vi "fp5YES.vi"   [LabVIEW 2016]
uses:
  <vilib>/NXT/Block Support/NXT_OutputPort.ctl
  <vilib>/NXT/Block Support/NXT_InputPort.ctl
  <vilib>/NXT/NXTIO Xnodes/NXTIONodeSubVIs/LEGOResetMotors.vi
  <vilib>/NXT/Dual Mode Library/Sensors/Touch_Released.vi
  <vilib>/NXT/Dual Mode Library/Sensors/EV3_Color_Reflect.vi
  <vilib>/NXT/NXTIO Xnodes/NXTIONodeSubVIs/NXTMoveMotors.vi
  <vilib>/NXT/NXTIO Xnodes/NXTIONodeSubVIs/NXTMotorRunDistance.vi
  <vilib>/NXT/NXTIO Xnodes/NXTIONodeSubVIs/NXTStopMotors.vi
  <vilib>/NXT/Dual Mode Library/Sound/PlayAsharp.vi
  <vilib>/NXT/Dual Mode Library/Sound/PlayC.vi
  <vilib>/NXT/Subs/LVHSConnector.ctl
  <vilib>/NXT/NXTIO Xnodes/AddressXNode/NXTIOAddress.xnode
  <vilib>/NXT/NXTIO Xnodes/NXTIOXNode/NXTIO.xnode
  <vilib>/NXT/LegoClasses/BrickReference/BrickReference.lvclass
types:
  T1 = typedef "NXT_OutputPort.ctl" = u8
  T2 = typedef "NXT_InputPort.ctl" = u32
  T3 = typedef "LVHSConnector.ctl" = refnum<class "BrickReference.lvclass">
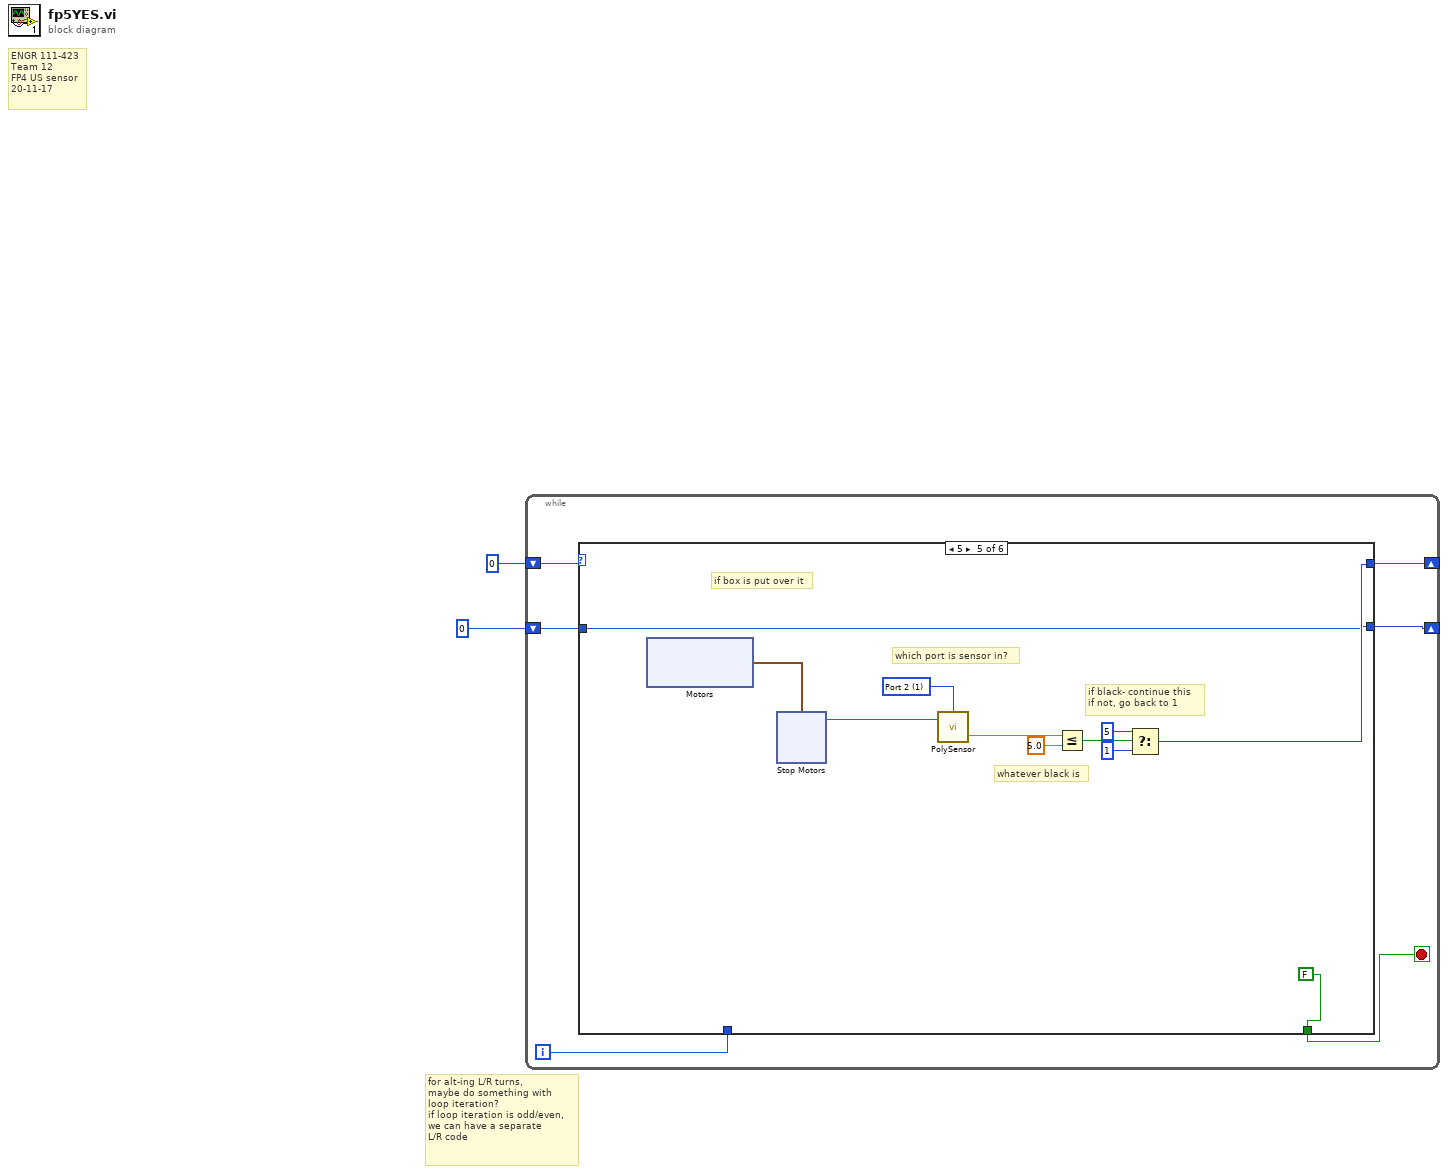
[diagram p0: block diagram]
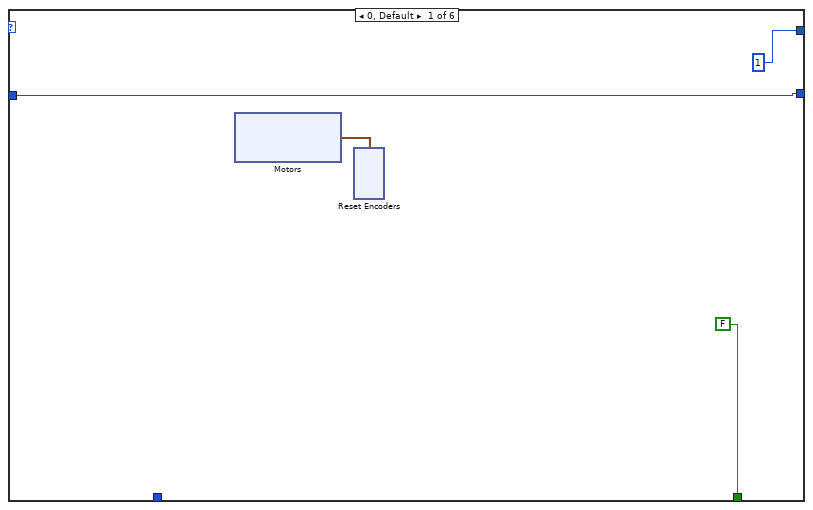
[diagram p2: hidden frame]
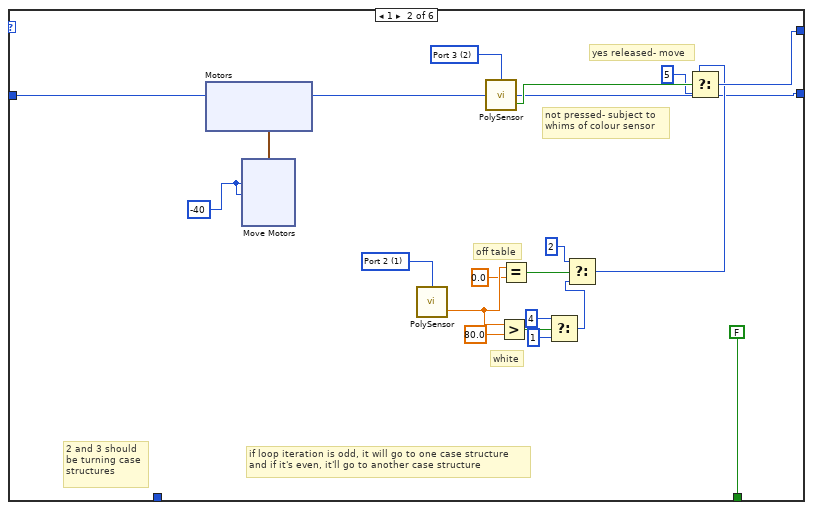
[diagram p3: hidden frame]
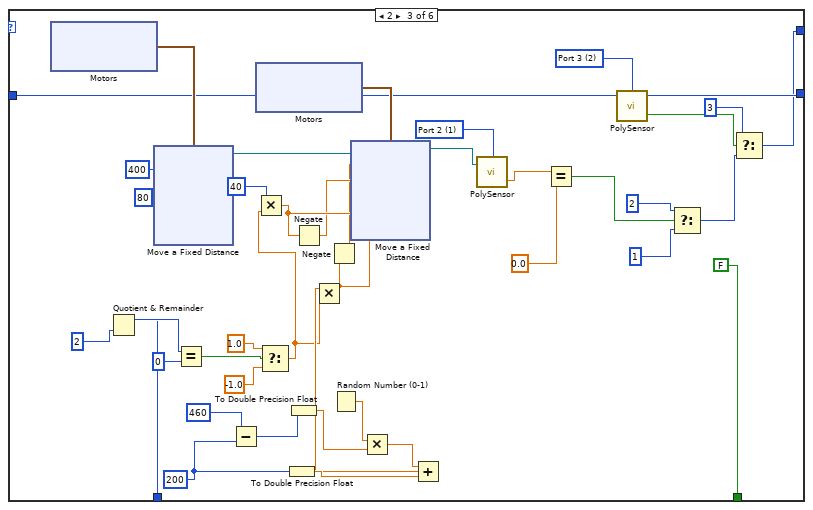
[diagram p4: hidden frame]
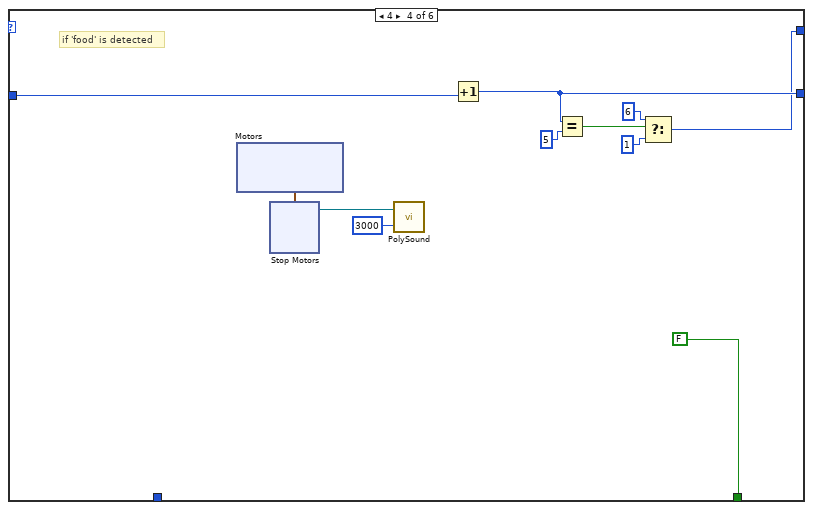
[diagram p5: hidden frame]
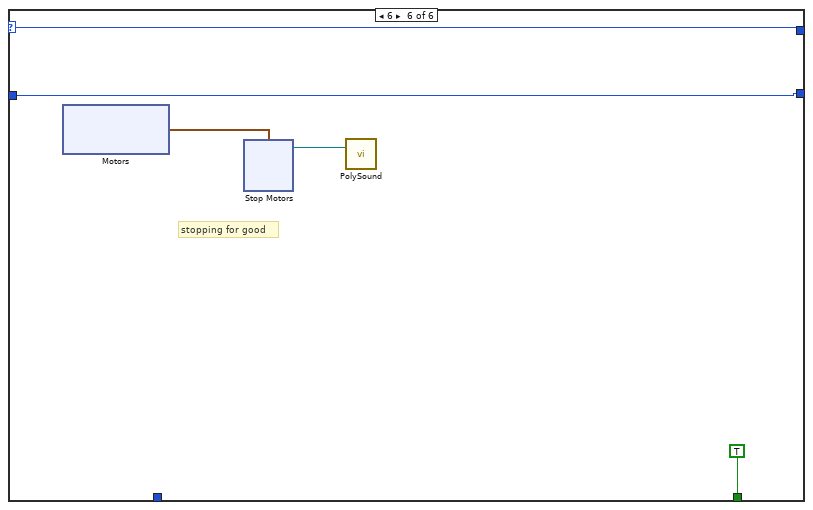
[diagram p6: hidden frame]
diagram:
  # "for alt-ing L/R turns,\nmaybe do something with\nloop iteration?\nif loop iteration is odd/even,\nwe can have a separate\nL/R code"
  # "ENGR 111-423\nTeam 12\nFP4 US sensor\n20-11-17"
  n1 = while {
    shift-right: [w6] -> _
    shift-left: 0 -> [w8]
    shift-right: [w4] -> _
    shift-left: 0 -> [w5]
    i -> [w3]
    stop <- w7 stop-if-true
    n2 = case shown="5" w8 {
      selector: w8 -> [_ _ _ _ _ w149]
      tunnel: [FALSE FALSE FALSE FALSE FALSE TRUE] -> w7
      tunnel: [1 w25 w56 w112 w131 w149] -> w6
      tunnel: w5 -> [w9 w19 w57 w119 w129 w146]
      tunnel: [w9 w19 w57 w116 w129 w146] -> w4
      tunnel: w3 -> [_ _ w58 _ _ _]
      frame 0, Default {
        n3 = xnode "Motors"() -> ("Motor"=w10:cluster{"Port":T1, "Port":T1})
        n4 = xnode "Reset Encoders"("Motors"=w10) -> ()  [unwired: 1 in, 1 out]
      }
      frame 1 {
        w26 = T2 1 items=["Port 1", "Port 2", "Port 3", "Port 4"] ("Port (Port 1)")
        w34 = T2 2 items=["Port 1", "Port 2", "Port 3", "Port 4"] ("Port (Port 1)")
        w35 = -40 ("Distance 1")
        # "white"
        # "off table"
        # "2 and 3 should\nbe turning case\nstructures"
        # "if loop iteration is odd, it will go to one case structure\nand if it's even, it'll go to another case structure"
        # "not pressed- subject to\nwhims of colour sensor"
        # "yes released- move"
        n5 = xnode "Motors"() -> ("Motor"=w36:cluster{"Port":T1, "Port":T1})
        n6 = xnode "Move Motors"("Power/Speed 2"=w35, "Power/Speed 1"=w35, "Motors"=w36) -> ()  [unwired: 1 in, 1 out]
        n7 = call-poly <vilib>:"PolySensor.vi"("Port (Port 1)"=w26) -> ("Scaled Value"=w27:sgl)  [unwired: 2 in, 1 out]
        n8 = call-poly <vilib>:"PolySensor.vi"("Port (Port 1)"=w34) -> ("Yes / No"=w33:bool)  [unwired: 2 in, 1 out]
        n9 = Greater?(x=w27, y=sgl 80.0) -> (0:w31:bool)
        n10 = Equal?(x=w27, y=sgl 0.0) -> (x = y?=w29:bool)
        n11 = Select(t=i16 4, s=w31, f=i16 1) -> (s? t:f=w23:i16)
        n12 = Select(t=2, s=w29, f=w23) -> (s? t:f=w20:i32)
        n13 = Select(t=w20, s=w33, f=i16 5 ("t")) -> (s? t:f=w25:i32)
      }
      frame 2 {
        w53 = 200
        w73 = 80 ("Distance 1")
        w74 = 400 ("Distance 1")
        w78 = T2 1 items=["Port 1", "Port 2", "Port 3", "Port 4"] ("Port (Port 1)")
        w80 = T2 2 items=["Port 1", "Port 2", "Port 3", "Port 4"] ("Port (Port 1)")
        n14 = xnode "Motors"() -> ("Motor"=w75:cluster{"Port":T1, "Port":T1})
        n15 = Quotient & Remainder(x=w58, y=2) -> (x-y*floor(x/y)=w65:i32)  [unwired: 1 out]
        n16 = xnode "Move a Fixed Distance"("Speed 2"=w73, "Speed 1"=w73, "Distance 2"=w74, "Distance 1"=w74, "Motors"=w75) -> ("NXT/EV3"=w72:T3)  [unwired: 1 in]
        n17 = Equal?(x=w65, y=0) -> (x = y?=w63:bool)
        n18 = Subtract(x=460, y=w53) -> (x-y=w54:i32)
        n19 = xnode "Motors"() -> ("Motor"=w76:cluster{"Port":T1, "Port":T1})
        n20 = Select(t=1.0, s=w63, f=-1.0) -> (s? t:f=w47:dbl)
        n21 = Multiply(x=40 ("Distance 1"), y=w47) -> (x*y=w68:dbl)
        n22 = To Double Precision Float(number=w53) -> (double precision float=w49:dbl)
        n23 = To Double Precision Float(number=w54) -> (double precision float=w52:dbl)
        n24 = Negate(x=w68) -> (-x=w67:dbl)
        n25 = Random Number (0-1)() -> (number: 0 to 1=w51:dbl)
        n26 = Multiply(x=w51, y=w52) -> (x*y=w50:dbl)
        n27 = Add(x=w50, y=w49) -> (x+y=w48:dbl)
        n28 = Multiply(x=w48, y=w47) -> (x*y=w46:dbl)
        n29 = Negate(x=w46) -> (-x=w60:dbl)
        n30 = xnode "Move a Fixed Distance"("Speed 2"=w68, "Speed 1"=w67, "Distance 2"=w46, "Distance 1"=w60, "Motors"=w76, "NXT/EV3"=w72) -> ("NXT/EV3"=w70:T3)
        n31 = call-poly <vilib>:"PolySensor.vi"("NXT/EV3"=w70, "Port (Port 1)"=w78) -> ("Scaled Value"=w77:sgl)  [unwired: 1 in, 1 out]
        n32 = Equal?(x=w77, y=0.0) -> (x = y?=w81:bool)
        n33 = call-poly <vilib>:"PolySensor.vi"("Port (Port 1)"=w80) -> ("Yes / No"=w79:bool)  [unwired: 2 in, 1 out]
        n34 = Select(t=2, s=w81, f=1) -> (s? t:f=w84:i32)
        n35 = Select(t=3, s=w79, f=w84) -> (s? t:f=w56:i32)
      }
      frame 4 {
        # "if 'food' is detected"
        n36 = xnode "Motors"() -> ("Motor"=w121:cluster{"Port":T1, "Port":T1})
        n37 = xnode "Stop Motors"("Motors"=w121) -> ("NXT/EV3"=w122:T3)  [unwired: 1 in]
        n38 = call-poly <vilib>:"PolySound.vi"("Duration (500 ms)"=u16 3000, "NXT/EV3"=w122) -> ()  [unwired: 2 in, 1 out]
        n39 = Increment(x=w119) -> (x+1=w116:i32)
        n40 = Equal?(x=w116, y=5) -> (x = y?=w117:bool)
        n41 = Select(t=6, s=w117, f=1) -> (s? t:f=w112:i32)
      }
      frame 5 {
        w137 = T2 1 items=["Port 1", "Port 2", "Port 3", "Port 4"] ("Port (Port 1)")
        # "if black- continue this\nif not, go back to 1"
        # "whatever black is"
        # "which port is sensor in?"
        # "if box is put over it"
        n42 = xnode "Motors"() -> ("Motor"=w139:cluster{"Port":T1, "Port":T1})
        n43 = xnode "Stop Motors"("Motors"=w139) -> ("NXT/EV3"=w138:T3)  [unwired: 1 in]
        n44 = call-poly <vilib>:"PolySensor.vi"("NXT/EV3"=w138, "Port (Port 1)"=w137) -> ("Scaled Value"=w136:sgl)  [unwired: 1 in, 1 out]
        n45 = Less Or Equal?(x=w136, y=sgl 5.0) -> (x <= y?=w134:bool)
        n46 = Select(t=i16 5, s=w134, f=i16 1) -> (s? t:f=w131:i16)
      }
      frame 6 {
        # "stopping for good"
        n47 = xnode "Motors"() -> ("Motor"=w150:cluster{"Port":T1, "Port":T1})
        n48 = xnode "Stop Motors"("Motors"=w150) -> ("NXT/EV3"=w147:T3)  [unwired: 1 in]
        n49 = call-poly <vilib>:"PolySound.vi"("NXT/EV3"=w147) -> ()  [unwired: 3 in, 1 out]
      }
    }
  }
